vi "Actor Core.vi"(8 "error in":errorcluster, 11 "Chat Window Model in":refnum<class "Chat Window Model.lvclass">) -> (0 "error out":errorcluster, 3 "Actor out":refnum<class "Actor.lvclass">)   [LabVIEW 2018, in "Chat Window Model.lvlib" / "Chat Window Model.lvclass"]
doc: "(<B>Filename</B>: Actor Framework.lvlib:Actor.lvclass:Actor Core.vi)\n\nReceives messages to the actor, reacts to them, and initiates any error handling that may shut the actor down.\n\nDescendant classes may override this VI to append parallel tasks for the actor to complete while it handles messages. Overrides use the Call Parent Method node."
uses:
  Chat Window Model.lvclass
  C:/Program Files (x86)/National Instruments/LabVIEW 2018/vi.lib/ActorFramework/Actor/Actor.lvclass
  <vilib>/ActorFramework/Actor/Actor.lvclass
  Chat Window Interface/Chat Window Interface.lvclass
  C:/Users/Thomas/Documents/YouTube Videos/Actor Oriented Design/10. Recap of Actor Core Overrides/Chat Room Actors/Chat Window UI Controller/Chat Window UI Controller/Chat Window UI Controller.lvclass
  Chat Window Model Messages/User Updated Status Msg/User Updated Status Msg.lvclass
  C:/Users/Thomas/Documents/YouTube Videos/Actor Oriented Design/10. Recap of Actor Core Overrides/Chat Room Actors/Chat Window UI Controller/Chat Window UI Controller Messages/Status Updated Msg/Status Updated Msg.lvclass
  Chat Window Model Messages/Forward Direct Message Msg/Forward Direct Message Msg.lvclass
  C:/Users/Thomas/Documents/YouTube Videos/Actor Oriented Design/10. Recap of Actor Core Overrides/Chat Room Actors/Chat Window UI Controller/Chat Window UI Controller Messages/Direct Message Msg/Direct Message Msg.lvclass
  Chat Window UI Controller/Chat Window UI Controller/Chat Window UI Controller.lvclass/Chat Window UI Controller.ctl
  Chat Window Model.lvclass/Chat Window Model.ctl
  Chat Window UI Controller/Chat Window UI Controller/Chat Window UI Controller.lvclass
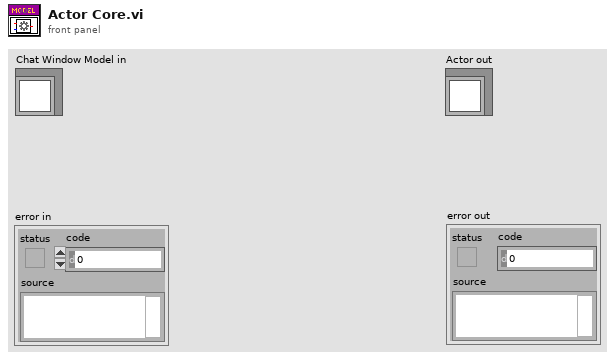
[diagram p1: front panel]
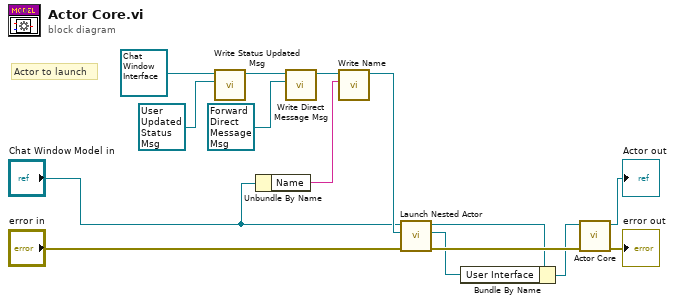
[diagram p0: block diagram]
diagram:
  # "Actor to launch"
  n1 = call "Write Status Updated Msg.vi"("Chat Window UI Controller.lvlib:Status Updated Msg.lvclass"=refnum<class "User Updated Status Msg.lvclass"> refnum ("Chat Window Model.lvlib:User Updated Status Msg.lvclass"), "Chat Window UI Controller in"=refnum<class "Chat Window Interface.lvclass"> refnum ("Chat Window Interface.lvlib:Chat Window Interface.lvclass")) -> ("Chat Window UI Controller out"=w6:refnum<class "Chat Window Interface.lvclass">)  [unwired: 9 in]
  n2 = Unbundle By Name("Chat Window Model in") -> ("Name"=w1:string)
  n3 = call "Write Direct Message Msg.vi"("Chat Window UI Controller.lvlib:Direct Message Msg.lvclass"=refnum<class "Forward Direct Message Msg.lvclass"> refnum ("Chat Window Model.lvlib:Forward Direct Message Msg.lvclass"), "Chat Window UI Controller in"=w6) -> ("Chat Window UI Controller out"=w4:refnum<class "Chat Window Interface.lvclass">)  [unwired: 9 in]
  n4 = call "Write Name.vi"("Name"=w1, "Chat Window UI Controller in"=w4) -> ("Chat Window UI Controller out"=w3:refnum<class "Chat Window Interface.lvclass">)  [unwired: 8 in, 1 out]
  n5 = call <vilib>:"Launch Nested Actor.vi"("error in (no error)"="error in", "Nested Actor"=w3, "Caller Actor in"="Chat Window Model in") -> ("error out"=w12:errorcluster, "Nested Actor's Enqueuer"=w9:refnum<class "Message Enqueuer.lvclass">, "Caller Actor out"=w10:refnum<class "Chat Window Model.lvclass">)  [unwired: 6 in]
  n6 = Bundle By Name(cluster=w10, "User Interface"=w9) -> (w11:refnum<class "Chat Window Model.lvclass">)
  n7 = call-parent "Actor Core.vi"("error in"=w12, "Actor in"=w11) -> ("error out"=→"error out":errorcluster, "Actor out"=→"Actor out":refnum<class "Actor.lvclass">)  [unwired: 8 in]
